vi "ABB Read Webdaq.vi"(6 "Webdaq Report":cluster{"Report":string, "Interval":string}={"Report"="Test_1", "Interval"="LastScan"}, 7 "error in":errorcluster, 8 "Temp Cal":dbl[][](array[numeric]), 9 "Simulate webdaq":bool, 10 "connection ID":refnum<k5>) -> (0 "error out":errorcluster, 1 "Scaling":dbl[](array[numeric]), 2 "Offset":dbl[](array[numeric]), 3 "Raw rdgs":dbl[](array[numeric]), 4 "Scaled readings":dbl[](array[numeric]), 5 "data out":string)   [LabVIEW 2009]
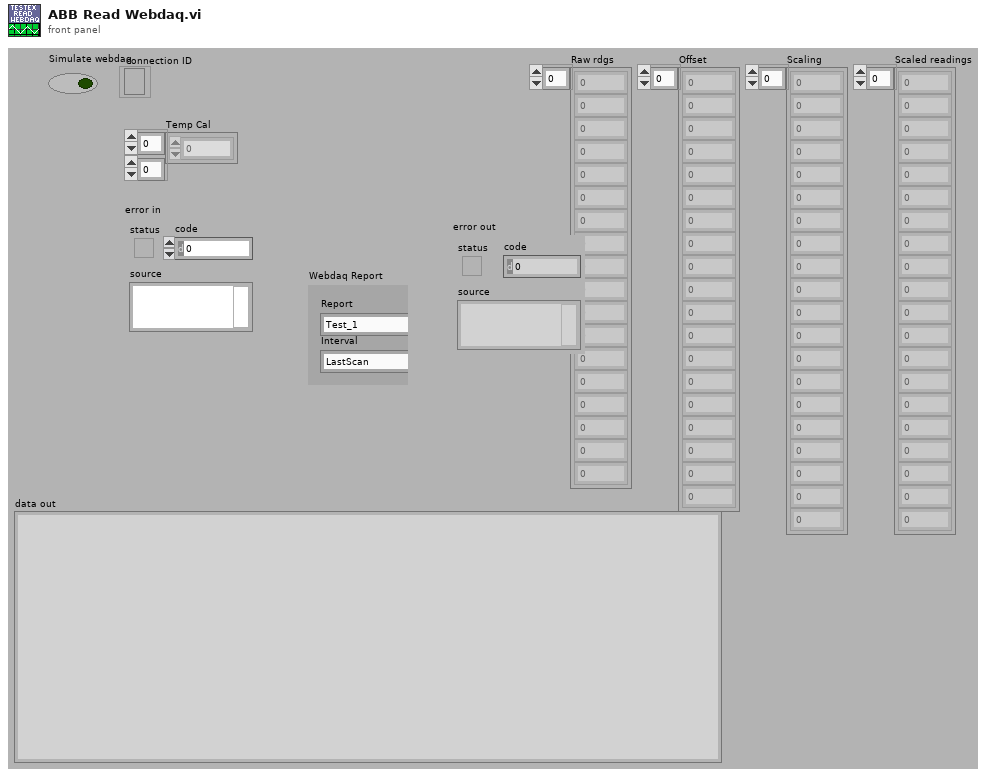
[diagram p1: front panel]
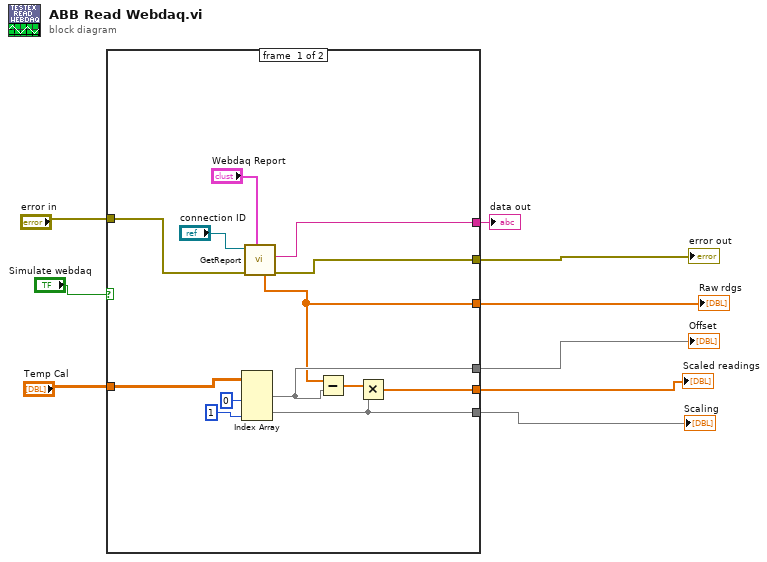
[diagram p0: block diagram]
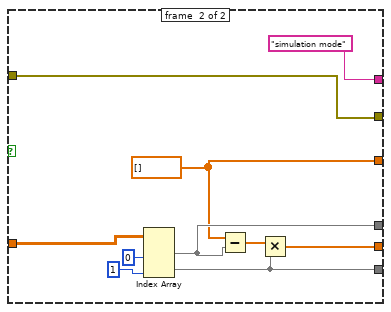
[diagram p2: hidden frame]
diagram:
  n1 = case shown="False" "Simulate webdaq" {
    tunnel: [w22 w32] -> w9
    tunnel: [w21 w31] -> w8
    tunnel: [w20 w30] -> w7
    tunnel: [w19 w24] -> w6
    tunnel: [w14 w25] -> w5
    tunnel: "Temp Cal" -> [w13 w26]
    tunnel: "error in" -> [w12 w25]
    tunnel: [w11 "simulation mode" ("data out")] -> w1
    frame #0 {
      n2 = Index Array(array=w13, index (col) #1=0 ("disabled index (col)"), index (col) #2=1 ("index (col)")) -> (element #1=w20:dbl[], element #2=w21:dbl[])  [unwired: 2 in]
      n3 = call "GetReport.vi"("Webdaq Report"="Webdaq Report", "error in"=w12, "connection ID"="connection ID") -> ("error out"=w14:errorcluster, "data out"=w11:string, "Averaged"=w19:dbl[])  [unwired: 4 in, 2 out]
      n4 = Subtract(x=w19, y=w20) -> (x-y=w18:dbl[])
      n5 = Multiply(x=w18, y=w21) -> (x*y=w22:dbl[])
    }
    frame #1 {
      w24 = dbl[] [] ("x")
      n6 = Index Array(array=w26, index (col) #1=0 ("disabled index (col)"), index (col) #2=1 ("index (col)")) -> (element #1=w30:dbl[], element #2=w31:dbl[])  [unwired: 2 in]
      n7 = Subtract(x=w24, y=w30) -> (x-y=w29:dbl[])
      n8 = Multiply(x=w29, y=w31) -> (x*y=w32:dbl[])
    }
  }
  "Scaled readings" <- w9
  "Scaling" <- w8
  "Offset" <- w7
  "Raw rdgs" <- w6
  "error out" <- w5
  "data out" <- w1
